vi "Write Address.vi"(8 "error in":errorcluster, 10 "newAdd":string, 11 "AlicatCommBank in":refnum<class "AlicatCommBank.lvclass">=refnum) -> (0 "error out":errorcluster, 3 "AlicatCommBank out":refnum<class "AlicatCommBank.lvclass">)   [LabVIEW 2014, in "Alicat.lvlib" / "AlicatCommBank.lvclass"]
doc: "Change the address on a Alicat device. This VI will only change the address if there is one device in the bank and the string length is one."
uses:
  AlicatCommBank.lvclass
  Alicat.lvclass
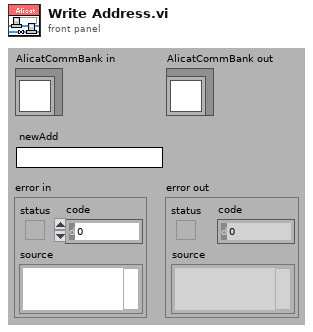
[diagram p1: front panel]
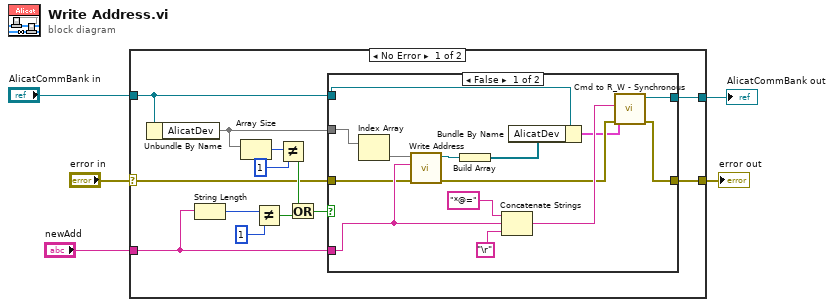
[diagram p0: block diagram]
diagram:
  n1 = case shown="No Error" "error in" {
    selector: "error in" -> [w9 w36]
    tunnel: [w8 w36] -> w4
    tunnel: [w6 w35] -> w2
    tunnel: "AlicatCommBank in" -> [w7 w35]
    tunnel: "newAdd" -> [w16 _]
    frame No Error {
      n2 = Unbundle By Name(w7) -> ("AlicatDev"=w10)
      n3 = String Length(string=w16) -> (length=w14:i32)
      n4 = Array Size(array=w10) -> (size(s)=w18:i32)
      n5 = Not Equal?(x=w14, y=1) -> (x != y?=w13:bool)
      n6 = Not Equal?(x=w18, y=1) -> (x != y?=w12:bool)
      n7 = Or(x=w12, y=w13) -> (x .or. y?=w11:bool)
      n8 = case shown="False" w11 {
        tunnel: w16 -> [w28 _]
        tunnel: w10 -> [w32 _]
        tunnel: w9 -> [w27 w34]
        tunnel: [w23 w34] -> w8
        tunnel: w7 -> [w22 w33]
        tunnel: [w19 w33] -> w6
        frame False {
          n9 = Index Array(array=w32) -> (element=w29)  [unwired: 1 in]
          n10 = call "Write Address.vi"("error in"=w27, "Address"=w28, "Alicat in"=w29) -> ("error out"=w24:errorcluster, "Alicat out"=w26:refnum<class "Alicat.lvclass">)  [unwired: 7 in]
          n11 = Build Array(w26) -> (w21:refnum<class "Alicat.lvclass">[])
          n12 = Concatenate Strings("*@=" ("string"), w28, "\r") -> (w25:string)
          n13 = Bundle By Name(cluster=w22, "AlicatDev"=w21) -> (w20:cluster{})
          n14 = call-dynamic "Cmd to R_W - Synchronous.vi"("error in"=w24, "write buffer"=w25, "Serial IO in"=w20) -> ("error out"=w23:errorcluster, "Serial IO out"=w19:refnum<class "AlicatCommBank.lvclass">)  [unwired: 6 in, 1 out]
        }
        frame True {
        }
      }
    }
    frame Error {
    }
  }
  "error out" <- w4
  "AlicatCommBank out" <- w2
